vi "TestingLoops.vi"   [LabVIEW 2012]
uses:
  <userlib>/Rogers RIO/URAPI/URAPI_Comparison.ctl
types:
  T1 = typedef "URAPI_Comparison.ctl" = enum16{">", "<", "=", "!="}
  T2 = typedef "URAPI_Control.ctl" = cluster{"Script":string, "Whiles":u8[], "Ifs":u8[], "remote":bool, "RIO Settings":T3, "Supress Err":bool}
  T3 = typedef "RIO_Control.ctl" = cluster{"IP Address":string, "Connected?":bool, "connection ID":refnum<k5>, "Script":string}
  T4 = typedef "URAPI_Control.ctl" = cluster{"Script":string, "Whiles":u8[], "Ifs":u8[], "Supress Err":bool, "Errors":string}
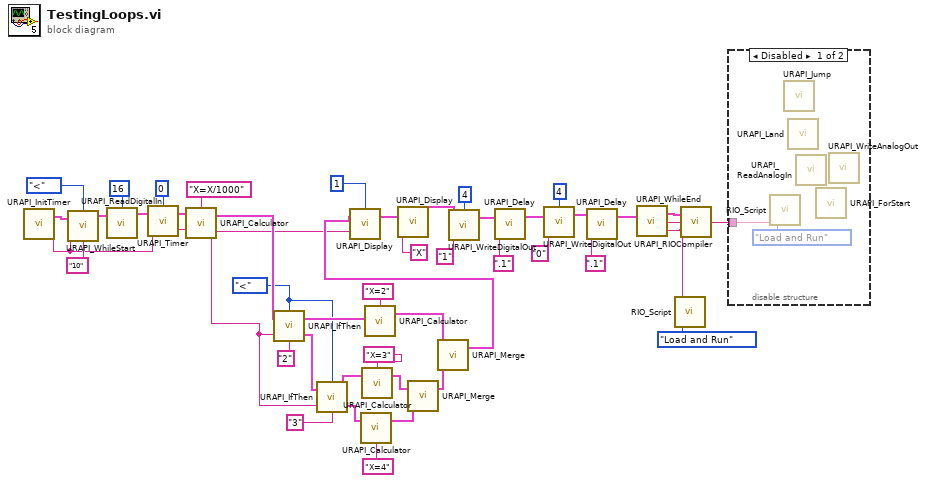
[diagram p0: block diagram]
diagram:
  w6 = URAPI_Comparison."<" ("Comparison")
  n1 = call <userlib>:"URAPI_InitTimer.vi"() -> ("Variable out"=w21:string, "URAPI Script out"=w24:T2)  [unwired: 4 in]
  n2 = call <userlib>:"URAPI_WhileStart.vi"("Variable In"=w21, "Compare to"="10", "URAPI Script"=w24, "Comparison"=URAPI_Comparison."<") -> ("URAPI Script Out"=w27:T2)  [unwired: 1 out]
  n3 = call <userlib>:"URAPI_ReadDigitalIn.vi"("URAPI Script"=w27, "Channel"=16) -> ("URAPI Script"=w28:T2)  [unwired: 2 in, 1 out]
  n4 = call <userlib>:"URAPI_Timer.vi"("Variable In"=w21, "URAPI Script"=w28, "Timer"=u8 0) -> ("Variable out"=w25:string, "URAPI Script out"=w26:T2)  [unwired: 1 in]
  n5 = call <userlib>:"URAPI_Calculator.vi"("X"=w25, "URAPI Script"=w26, "Formula"="X=X/1000") -> ("Variable Out"=w1:string, "URAPI Script"=w9:T2)  [unwired: 1 in]
  n6 = call <userlib>:"URAPI_IfThen.vi"("Variable In"=w1, "Compare to"="2", "URAPI Script"=w9, "Comparison"=w6) -> ("URAPI False"=w20:T2, "URAPI True"=w18:T2)
  n7 = call <userlib>:"URAPI_IfThen.vi"("Variable In"=w1, "Compare to"="3", "URAPI Script"=w20, "Comparison"=w6) -> ("URAPI False"=w15:T2, "URAPI True"=w13:T2)
  n8 = call <userlib>:"URAPI_Calculator.vi"("URAPI Script"=w15, "Formula"="X=4") -> ("URAPI Script"=w14:T2)  [unwired: 2 in, 1 out]
  n9 = call <userlib>:"URAPI_Calculator.vi"("URAPI Script"=w13, "Formula"="X=3") -> ("URAPI Script"=w16:T2)  [unwired: 2 in, 1 out]
  n10 = call <userlib>:"URAPI_Calculator.vi"("URAPI Script"=w18, "Formula"="X=2") -> ("URAPI Script"=w10:T2)  [unwired: 2 in, 1 out]
  n11 = call <userlib>:"URAPI_Merge.vi"("URAPI False"=w14, "URAPI True"=w16) -> ("URAPI Script"=w19:T2)  [unwired: 3 in]
  n12 = call <userlib>:"URAPI_Merge.vi"("URAPI False"=w19, "URAPI True"=w10) -> ("URAPI Script"=w4:T2)  [unwired: 3 in]
  n13 = call <userlib>:"URAPI_Display.vi"("Variable In"=w1, "URAPI Script"=w4, "Line"=1) -> ("URAPI Script"=w2:T2)  [unwired: 1 in, 1 out]
  n14 = call <userlib>:"URAPI_Display.vi"("Variable In"="X", "URAPI Script"=w2) -> ("URAPI Script"=w35:T2)  [unwired: 2 in, 1 out]
  n15 = call <userlib>:"URAPI_WriteDigitalOut.vi"("Variable In"="1", "URAPI Script"=w35, "Channel"=4) -> ("URAPI Script"=w39:T4)  [unwired: 1 in, 1 out]
  n16 = call <userlib>:"URAPI_Delay.vi"("Variable In"=".1" ("Compare to"), "URAPI Script"=w39) -> ("URAPI Script out"=w38:T4)  [unwired: 3 in]
  n17 = call <userlib>:"URAPI_WriteDigitalOut.vi"("Variable In"="0", "URAPI Script"=w38, "Channel"=4) -> ("URAPI Script"=w36:T4)  [unwired: 1 in, 1 out]
  n18 = call <userlib>:"URAPI_Delay.vi"("Variable In"=".1" ("Compare to"), "URAPI Script"=w36) -> ("URAPI Script out"=w34:T4)  [unwired: 3 in]
  n19 = call <userlib>:"URAPI_WhileEnd.vi"("URAPI Script"=w34) -> ("URAPI Script Out"=w33:T4)  [unwired: 4 in]
  n20 = call <userlib>:"URAPI_RIOCompiler.vi"("URAPI Script"=w33) -> ("Script"=w32:string)  [unwired: 4 in]
  n21 = call <userlib>:"RIO_Script.vi"("Execution Mode"=enum16{"Load", "Run", "Load and Run"}."Load and Run", "Script"=w32) -> ()  [unwired: 2 in, 1 out]
  n22 = disable-structure shown="Disabled" {
    disable-tunnel: w32 -> [w47 _]
    frame Disabled {
      n23 = call <userlib>:"RIO_Script.vi"("Execution Mode"=enum16{"Load", "Run", "Load and Run"}."Load and Run", "Script"=w47) -> ()  [unwired: 2 in, 1 out]
      n24 = call <userlib>:"URAPI_Jump.vi"() -> ()  [unwired: 5 in, 1 out]
      n25 = call <userlib>:"URAPI_Land.vi"() -> ()  [unwired: 5 in, 1 out]
      n26 = call <userlib>:"URAPI_ReadAnalogIn.vi"() -> ()  [unwired: 4 in, 2 out]
      n27 = call <userlib>:"URAPI_ForStart.vi"() -> ()  [unwired: 4 in, 2 out]
      n28 = call <userlib>:"URAPI_WriteAnalogOut.vi"() -> ()  [unwired: 4 in, 2 out]
    }
    frame Enabled {
    }
  }
